vi "svc_Unit Label Manipulation.vi"(5 "operation":enum16{"Square (X^2)", "Divide (X/Y)"}(ring), 6 "Y unit label":string, 7 "X unit label":string) -> (3 "resulting unit label":string)   [LabVIEW 2017]
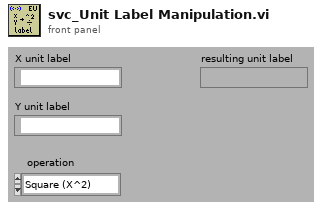
[diagram p1: front panel]
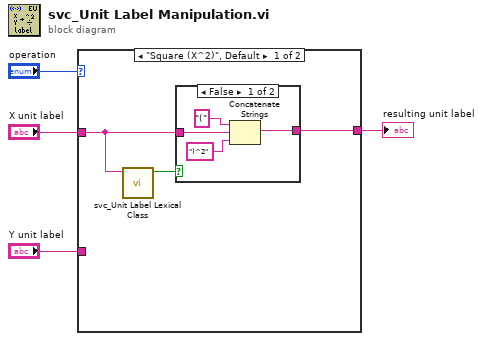
[diagram p0: block diagram]
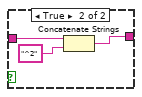
[diagram p2: hidden frame]
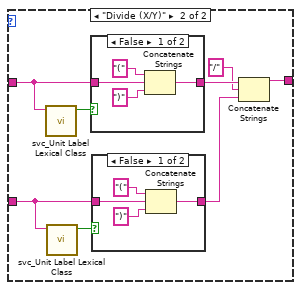
[diagram p3: hidden frame]
diagram:
  n1 = case shown="\"Square (X^2)\", Default" "operation" {
    tunnel: "X unit label" -> [w6 w18]
    tunnel: [w7 w21] -> w3
    tunnel: "Y unit label" -> [_ w16]
    frame "Square (X^2)", Default {
      n2 = call <vilib>:"svc_Unit Label Lexical Class.vi"("unit label"=w6) -> ("letters only?"=w5:bool)  [unwired: 6 in]
      n3 = case shown="False" w5 {
        tunnel: w6 -> [w11 w14]
        tunnel: [w8 w12] -> w7
        frame False {
          n4 = Concatenate Strings("(", w11, ")^2") -> (w8:string)
        }
        frame True {
          n5 = Concatenate Strings(w14, "^2") -> (w12:string)
        }
      }
    }
    frame "Divide (X/Y)" {
      n6 = call <vilib>:"svc_Unit Label Lexical Class.vi"("unit label"=w18) -> ("letters only?"=w17:bool)  [unwired: 6 in]
      n7 = call <vilib>:"svc_Unit Label Lexical Class.vi"("unit label"=w16) -> ("letters only?"=w15:bool)  [unwired: 6 in]
      n8 = case shown="False" w17 {
        tunnel: w18 -> [w31 w32]
        tunnel: [w28 w32] -> w22
        frame False {
          n9 = Concatenate Strings("(", w31, ")") -> (w28:string)
        }
        frame True {
        }
      }
      n10 = case shown="False" w15 {
        tunnel: w16 -> [w26 w27]
        tunnel: [w23 w27] -> w20
        frame False {
          n11 = Concatenate Strings("(", w26, ")") -> (w23:string)
        }
        frame True {
        }
      }
      n12 = Concatenate Strings(w22, "/" ("Y unit label"), w20) -> (w21:string)
    }
  }
  "resulting unit label" <- w3
